vi "Auto generate POIs.vi"(10 "Number of POI to generate":i32, 11 "Image refnum in":T3) -> (2 "POI Array":T1[](array[typedef]) {"Zoom" min=1.0 max=10.0 step=0.10000000149011612}, 3 "Number of POI generated":i32)   [LabVIEW 2017]
uses:
  <vilib>/vision/Image Controls.llb/IMAQ Image.ctl
  Typedefs/ROI spec.ctl
  Typedefs/ROI ID Enum.ctl
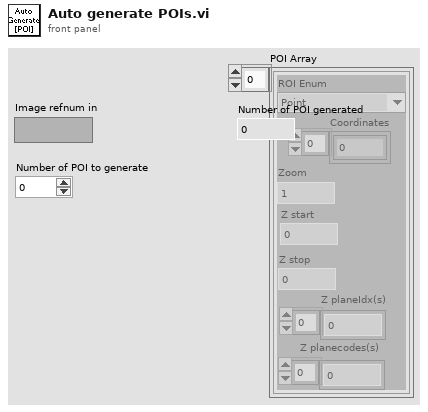
[diagram p1: front panel]
types:
  T1 = typedef "ROI spec.ctl" = cluster{"Coordinates":i32[], "Zoom":dbl, "ROI Enum":T2, "Z planeIdx(s)":i32[], "Z planecodes(s)":u8[], "Z start":dbl, "Z stop":dbl}
  T2 = typedef "ROI ID Enum.ctl" = enum16{"Point", "MiniScan", "Comp. MiniScan", "Rectangle", "Comp. volume", "Arb. plane point"}
  T3 = typedef "IMAQ Image.ctl" = refnum<image>
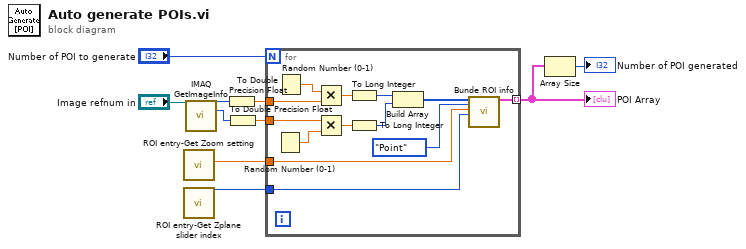
[diagram p0: block diagram]
diagram:
  n1 = call "ROI entry-Get Zoom setting.vi"() -> ("Zoom Value"=w2:dbl)  [unwired: 9 in, 2 out]
  n2 = call "ROI entry-Get Zplane slider index.vi"() -> ("Z-plane slider's index (zero-based)"=w1:i32)  [unwired: 10 in, 1 out]
  n3 = call "IMAQ GetImageInfo"("Image"="Image refnum in") -> ("Y Resolution"=w8:i32, "X Resolution"=w9:i32)  [unwired: 3 in, 6 out]
  n4 = To Double Precision Float(number=w9) -> (double precision float=w4:dbl)
  n5 = To Double Precision Float(number=w8) -> (double precision float=w5:dbl)
  n6 = for {
    N: "Number of POI to generate" -> [_]
    tunnel: w4 -> [w21]
    tunnel: w5 -> [w20]
    tunnel: [w14] -> w6 mode=indexing
    tunnel: w2 -> [w13]
    tunnel: w1 -> [w11]
    n7 = Random Number (0-1)() -> (number: 0 to 1=w22:dbl)
    n8 = Random Number (0-1)() -> (number: 0 to 1=w23:dbl)
    n9 = Multiply(x=w23, y=w21) -> (x*y=w19:dbl)
    n10 = Multiply(x=w20, y=w22) -> (x*y=w17:dbl)
    n11 = To Long Integer(number=w19) -> (32bit integer=w18:i32)
    n12 = To Long Integer(number=w17) -> (32bit integer=w16:i32)
    n13 = Build Array(w18, w16) -> (w15:i32[])
    n14 = call "Bunde ROI info.vi"("ROI Coordinates"=w15, "ROI Enum"=ROI_ID_Enum."Point", "Zoom"=w13, "ZplaneIndex"=w11) -> ("ROI Info"=w14:T1)  [unwired: 15 in]
  }
  "POI Array" <- w6
  n15 = Array Size(array=w6) -> (size(s)=→"Number of POI generated":i32)
